vi "ITCHe3_Save_Info.vi"(8 "error in":errorcluster, 11 "Instrument parameters":T1) -> (0 "error out":errorcluster, 2 "Info array":string[][](array[string]), 3 "Instrument parameters out":T1)   [LabVIEW 2025]
uses:
  TYPE DEFS/S2DS_Instrument parameters.ctl
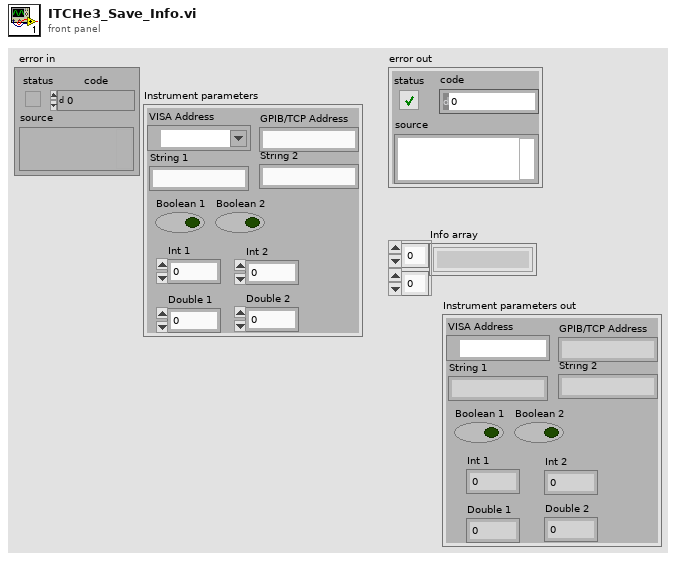
[diagram p1: front panel]
types:
  T1 = typedef "S2DS_Instrument parameters.ctl" = cluster{"VISA Address":refnum<visa-resource-name>, "GPIB/TCP Address":string, "String 1":string, "String 2":string, "Boolean 1":bool, "Boolean 2":bool, "Int 1":i32, "Int 2":i32, "Double 1":dbl, "Double 2":dbl}
  T2 = enum16{"Setpoint", "Sensor 1", "Sensor 2", "Sensor 3", "Temperature Error", "Heater Output (%)", "Heater Output (V)", "Gas Flow Output", "P Term", "I term", "D term", "Channel 1 Frequency/4", "Channel 2 Frequency/4", "Channel 3 Frequency/4"}
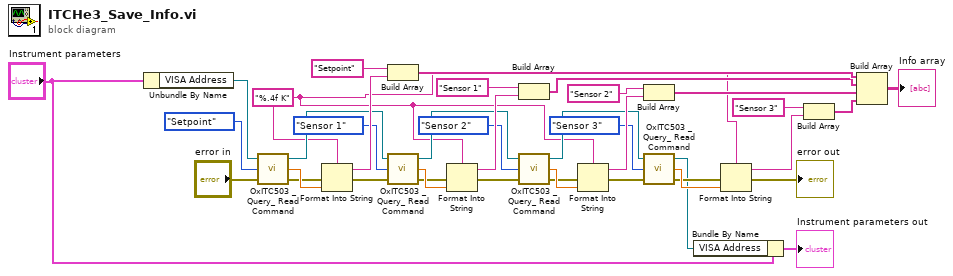
[diagram p0: block diagram]
diagram:
  w1 = "%.4f K"
  n1 = Unbundle By Name("Instrument parameters") -> ("VISA Address"=w5:refnum<visa-resource-name>)
  n2 = call "OxITC503 _Query_ Read Command.vi"("error in"="error in", "Read Item"=T2."Setpoint", "VISA session"=w5) -> ("error out (no error)"=w37:errorcluster, "Output of Read"=w38:dbl, "VISA session"=w18:refnum<visa-resource-name>)
  n3 = Format Into String(format string=w1, error in=w37, w38) -> (resulting string=w35:string, error out=w15:errorcluster)  [unwired: 1 in]
  n4 = Build Array("Setpoint" ("element"), w35) -> (w10:string[])
  n5 = call "OxITC503 _Query_ Read Command.vi"("error in"=w15, "Read Item"=T2."Sensor 1", "VISA session"=w18) -> ("error out (no error)"=w32:errorcluster, "Output of Read"=w33:dbl, "VISA session"=w17:refnum<visa-resource-name>)
  n6 = Format Into String(format string=w1, error in=w32, w33) -> (resulting string=w30:string, error out=w14:errorcluster)  [unwired: 1 in]
  n7 = Build Array("Sensor 1" ("element"), w30) -> (w9:string[])
  n8 = call "OxITC503 _Query_ Read Command.vi"("error in"=w14, "Read Item"=T2."Sensor 2", "VISA session"=w17) -> ("error out (no error)"=w27:errorcluster, "Output of Read"=w28:dbl, "VISA session"=w16:refnum<visa-resource-name>)
  n9 = Format Into String(format string=w1, error in=w27, w28) -> (resulting string=w25:string, error out=w13:errorcluster)  [unwired: 1 in]
  n10 = Build Array("Sensor 2" ("element"), w25) -> (w8:string[])
  n11 = call "OxITC503 _Query_ Read Command.vi"("error in"=w13, "Read Item"=T2."Sensor 3", "VISA session"=w16) -> ("error out (no error)"=w22:errorcluster, "Output of Read"=w23:dbl, "VISA session"=w3:refnum<visa-resource-name>)
  n12 = Bundle By Name(cluster="Instrument parameters", "VISA Address"=w3) -> (→"Instrument parameters out":T1)
  n13 = Format Into String(format string=w1, error in=w22, w23) -> (resulting string=w20:string, error out=→"error out":errorcluster)  [unwired: 1 in]
  n14 = Build Array("Sensor 3" ("element"), w20) -> (w7:string[])
  n15 = Build Array(w10, w9, w8, w7) -> (→"Info array":string[][])
